vi "Set Cooler Power Status.vi"(8 "error in (no error)":errorcluster, 11 "CCDCamera in":refnum<class "iKon-L.lvclass">) -> (0 "error out":errorcluster, 3 "CCDCamera out":refnum<class "iKon-L.lvclass">)   [LabVIEW 2018, in "iKon-L.lvclass"]
doc: "Turn the cooler on or off"
uses:
  iKon-L.lvclass
  C:/Users/Denis/Desktop/S4ACS/S4ACS/Sim_CCD/Sim_CCD.lvclass
  Sim_CCD/Sim_CCD.lvclass
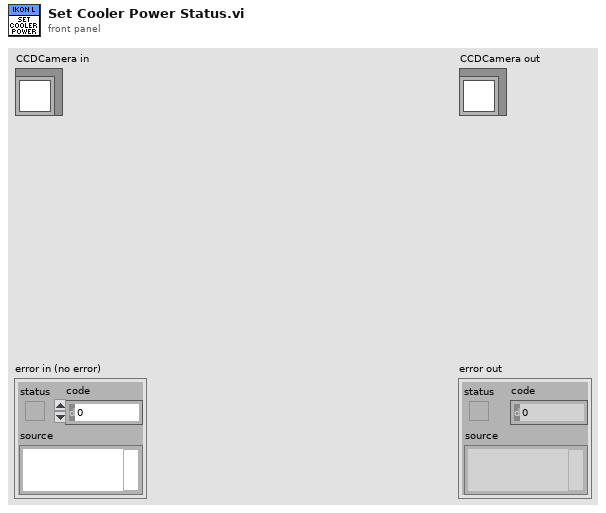
[diagram p1: front panel]
types:
  T1 = cluster{"EXPTIME":dbl, "#FRAMES":u32, "COOLER_POWER_STATUS":u16, "TEMP":i32}
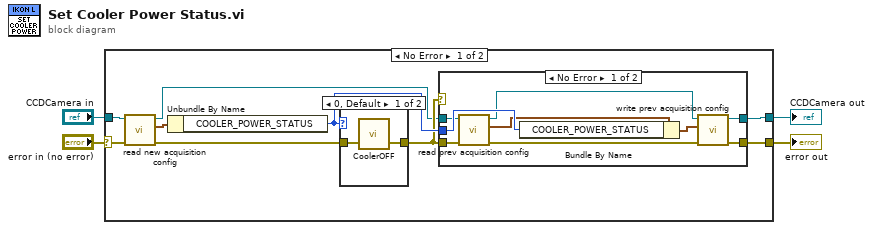
[diagram p0: block diagram]
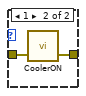
[diagram p3: hidden frame]
diagram:
  n1 = case shown="No Error" "error in (no error)" {
    selector: "error in (no error)" -> [w8 w29]
    tunnel: "CCDCamera in" -> [w9 w30]
    tunnel: [w12 w30] -> w2
    tunnel: [w13 w29] -> w1
    frame No Error {
      n2 = call "read new acquisition config.vi"("error in (no error)"=w8, "Simulated_CCD_Camera in"=w9) -> ("error out"=w6:errorcluster, "new acquisition configuration"=w7:T1, "Simulated_CCD_Camera out"=w5:refnum<class "iKon-L.lvclass">)  [unwired: 7 in]
      n3 = Unbundle By Name(w7) -> ("COOLER_POWER_STATUS"=w11:u16)
      n4 = case shown="0, Default" w11 {
        tunnel: [w26 w28] -> w10
        tunnel: w6 -> [w25 w27]
        frame 0, Default {
          n5 = call <userlib>:"CoolerOFF.vi"("error in (no error)"=w25) -> ("error out"=w26:errorcluster)  [unwired: 1 in, 1 out]
        }
        frame 1 {
          n6 = call <userlib>:"CoolerON.vi"("error in (no error)"=w27) -> ("error out"=w28:errorcluster)  [unwired: 1 in, 1 out]
        }
      }
      n7 = case shown="No Error" w10 {
        tunnel: [w18 w24] -> w12
        tunnel: [w17 w23] -> w13
        tunnel: w5 -> [w21 w24]
        tunnel: w10 -> [w20 w23]
        tunnel: w11 -> [w22 _]
        frame No Error {
          n8 = call "read prev acquisition config.vi"("error in (no error)"=w20, "Simulated_CCD_Camera in"=w21) -> ("error out"=w15:errorcluster, "prev acquisition configuration"=w19:T1, "Simulated_CCD_Camera out"=w16:refnum<class "iKon-L.lvclass">)  [unwired: 7 in]
          n9 = Bundle By Name(cluster=w19, "COOLER_POWER_STATUS"=w22) -> (w14:T1)
          n10 = call "write prev acquisition config.vi"("error in (no error)"=w15, "prev acquisition configuration"=w14, "Simulated_CCD_Camera in"=w16) -> ("error out"=w17:errorcluster, "Simulated_CCD_Camera out"=w18:refnum<class "iKon-L.lvclass">)  [unwired: 7 in]
        }
        frame Error {
        }
      }
    }
    frame Error {
    }
  }
  "error out" <- w1
  "CCDCamera out" <- w2
